vi "Named Loggers.vi"() -> ()   [LabVIEW 2020]
uses:
  Source/LV Logging.lvlib
  Source/Type Defs/Debug Level.ctl
panel:
  in  "Debug Level in":T1
  out "error out":errorcluster
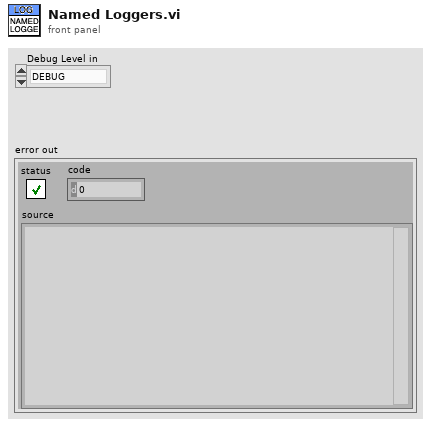
[diagram p1: front panel]
types:
  T1 = typedef "LV Logging.lvlib/Debug Level.ctl" = enum16{"DEBUG", "INFO", "WARN", "ERROR", "FATAL"}
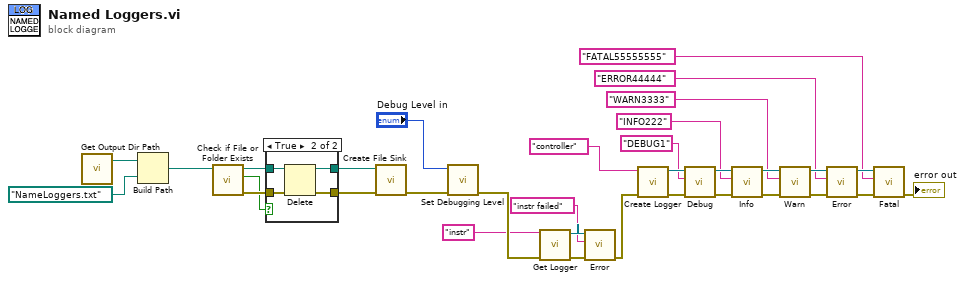
[diagram p0: block diagram]
diagram:
  n1 = call "Get Output Dir Path.vi"() -> ("Example/Output/ Dir"=w30:path)  [unwired: 3 in]
  n2 = Build Path(base path=w30, name or relative path=path "NameLoggers.txt") -> (appended path=w26:path)
  n3 = call <vilib>:"Check if File or Folder Exists.vi"("path"=w26) -> ("error out"=w24:errorcluster, "file or folder exists?"=w23:bool, "dup path"=w25:path)  [unwired: 8 in]
  n4 = case shown="True" w23 {
    tunnel: [w34 w39] -> w28
    tunnel: [w35 w38] -> w27
    tunnel: w25 -> [w35 w37]
    tunnel: w24 -> [w34 w36]
    frame False {
    }
    frame True {
      n5 = Delete(path (use dialog)=w37, error in=w36) -> (deleted path=w38:path, error out=w39:errorcluster)  [unwired: 3 in, 1 out]
    }
  }
  n6 = call "Create File Sink.vi"("error in (no error)"=w28, "Path"=w27) -> ("error out"=w32:errorcluster)  [unwired: 9 in]
  n7 = call "Set Debugging Level.vi"("error in (no error)"=w32, "Debug Level in"="Debug Level in") -> ("error out"=w22:errorcluster)  [unwired: 9 in]
  n8 = call "Get Logger.vi"("error in (no error)"=w22, "Name"="instr") -> ("error out"=w4:errorcluster, "Logger out"=w3:refnum<class "Logger.lvclass">)  [unwired: 8 in]
  n9 = call "Error.vi"("error in (no error)"=w4, "Log Text"="instr failed", "Logger in"=w3) -> ("error out"=w2:errorcluster)  [unwired: 7 in, 1 out]
  n10 = call "Create Logger.vi"("error in (no error)"=w2, "Name"="controller") -> ("error out"=w20:errorcluster, "Logger out"=w19:refnum<class "Logger.lvclass">)  [unwired: 8 in]
  n11 = call "Debug.vi"("error in (no error)"=w20, "Log Text"="DEBUG1", "Logger in"=w19) -> ("error out"=w17:errorcluster, "Logger out"=w18:refnum<class "Logger.lvclass">)  [unwired: 7 in]
  n12 = call "Info.vi"("error in (no error)"=w17, "Log Text"="INFO222", "Logger in"=w18) -> ("error out"=w16:errorcluster, "Logger out"=w15:refnum<class "Logger.lvclass">)  [unwired: 7 in]
  n13 = call "Warn.vi"("error in (no error)"=w16, "Log Text"="WARN3333", "Logger in"=w15) -> ("error out"=w13:errorcluster, "Logger out"=w14:refnum<class "Logger.lvclass">)  [unwired: 7 in]
  n14 = call "Error.vi"("error in (no error)"=w13, "Log Text"="ERROR44444", "Logger in"=w14) -> ("error out"=w12:errorcluster, "Logger out"=w11:refnum<class "Logger.lvclass">)  [unwired: 7 in]
  n15 = call "Fatal.vi"("error in (no error)"=w12, "Log Text"="FATAL55555555", "Logger in"=w11) -> ("error out"=→"error out":errorcluster)  [unwired: 7 in, 1 out]
